vi "GetMainSequence.vi"(6 "Stepnum":i32, 8 "error in (no error)":errorcluster, 11 "Compiler Settings":T1={"Python Path"=path "", "Main File"="mainscript.py", "Meta File"="metascript.txt", "Aux File"="auxscript.py", "Pre File"="metascript.txt"}) -> (0 "error out":errorcluster, 3 "Main pulse":T2)   [LabVIEW 2019]
uses:
  PulseControl.ctl
  Compiler/Params.ctl
  PulseCompiler/CompilerSettings.ctl
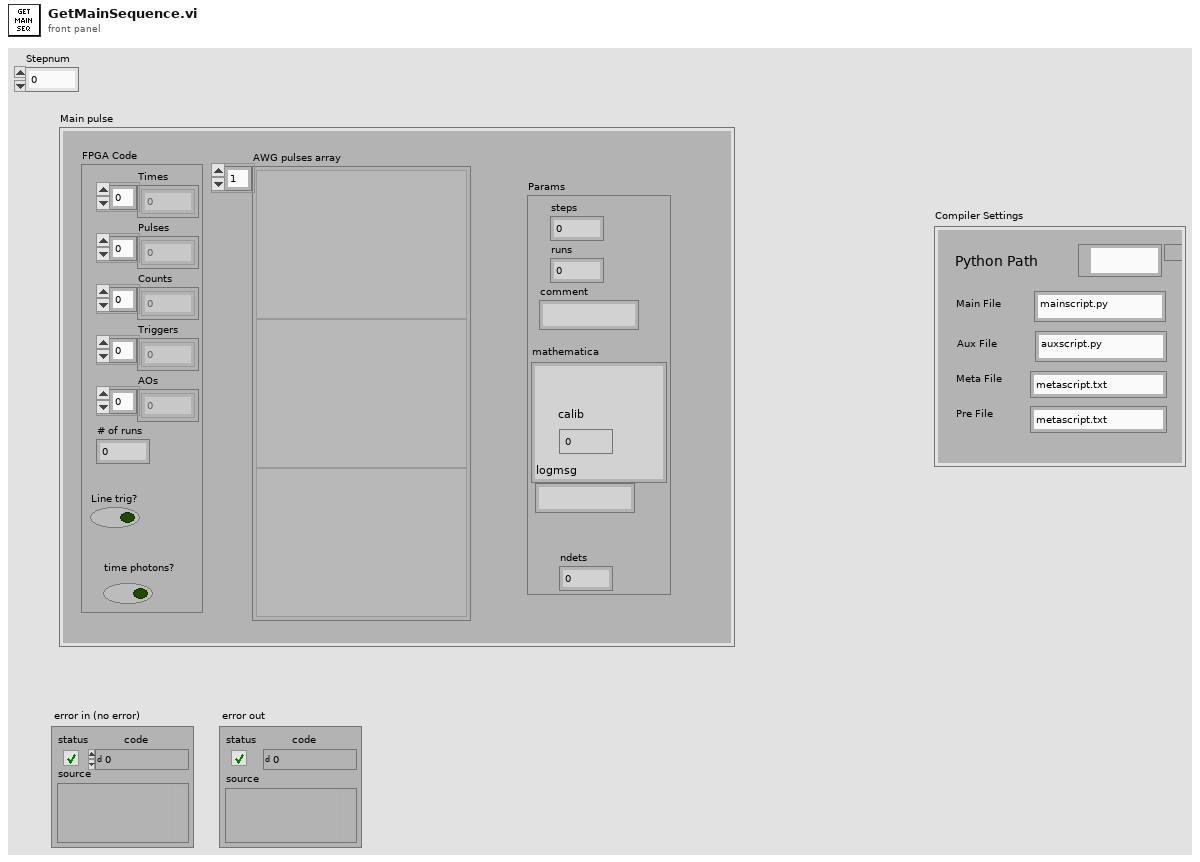
[diagram p1: front panel]
types:
  T1 = typedef "CompilerSettings.ctl" = cluster{"Python Path":path, "Main File":string, "Meta File":string, "Aux File":string, "Pre File":string}
  T2 = typedef "PulseControl.ctl" = cluster{"FPGA Code":cluster{"Times":u32[], "Pulses":u64[], "Counts":u8[], "Triggers":u8[], "AOs":u8[], "# of runs":i32, "Line trig?":bool, "time photons?":bool}, "AWG pulses array":variant[], "Params":T3}
  T3 = typedef "Params.ctl" = cluster{"steps":i16, "runs":i16, "comment":string, "mathematica":string, "calib":i8, "logmsg":string, "ndets":i16}
  T4 = typedef "SinglePulse.ctl" = cluster{"enabled":bool, "string":string, "time":dbl, "step":dbl, "dio":dbl, "count":dbl, "trigger":dbl, "AO":dbl}
  T5 = cluster{u32[], dbl[], "Count":dbl[], dbl[], dbl[], "# of runs":i32, "Line trig":bool, "save photon times":bool}
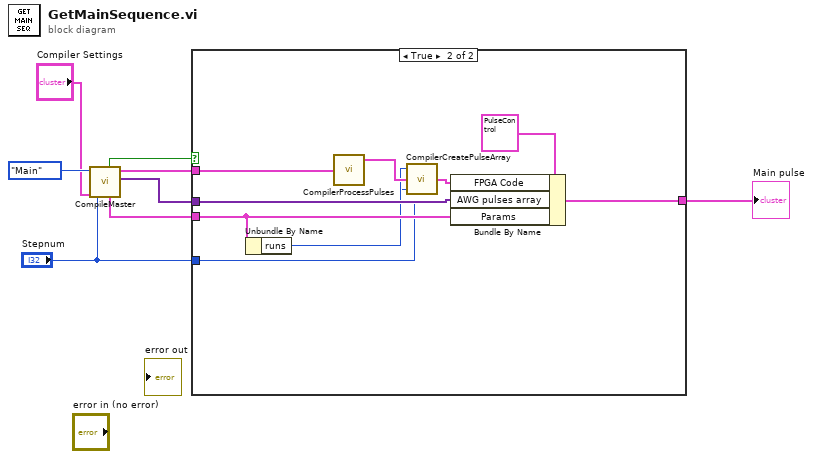
[diagram p0: block diagram]
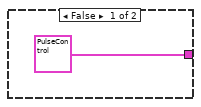
[diagram p2: hidden frame]
diagram:
  n1 = call "CompileMaster.vi"("Type"=enum16{"Meta", "Aux", "Main"}."Main" ("Enum"), "Stepnum"="Stepnum", "Compiler Settings"="Compiler Settings") -> ("CompileSuccess?"=w8:bool, "Params"=w7:T3, "PulseList"=w5:T4[], "RF Array"=w4:variant[])  [unwired: 1 in, 2 out]
  n2 = case shown="True" w8 {
    tunnel: [T2 {"FPGA Code"={"Times"=[], "Pulses"=[], "Counts"=[], "Triggers"=[], "AOs"=[], "# of runs"=0, "Line trig?"=FALSE, "time photons?"=FALSE}, "AWG pulses array"=[], "Params"={"steps"=0, "runs"=0, "comment"="", "mathematica"="", "calib"=0, "logmsg"="", "ndets"=0}} ("Pulse") w18] -> w3
    tunnel: w4 -> [_ w17]
    tunnel: w5 -> [_ w14]
    tunnel: w7 -> [_ w13]
    tunnel: "Stepnum" -> [_ w10]
    frame False {
    }
    frame True {
      n3 = Unbundle By Name(w13) -> ("runs"=w12:i16)
      n4 = call "CompilerProcessPulses.vi"("Pulse Seq In"=w14) -> ("Pulse Seq Out"=w16:T4[])  [unwired: 2 out]
      n5 = call "CompilerCreatePulseArray.vi"("step #"=w10, "Pulse Seq In"=w16, "runs"=w12) -> ("Pulse Seq Out"=w15:T5)
      n6 = Bundle By Name(cluster=T2 {"FPGA Code"={"Times"=[], "Pulses"=[], "Counts"=[], "Triggers"=[], "AOs"=[], "# of runs"=0, "Line trig?"=FALSE, "time photons?"=FALSE}, "AWG pulses array"=[], "Params"={"steps"=0, "runs"=0, "comment"="", "mathematica"="", "calib"=0, "logmsg"="", "ndets"=0}} ("Aux Pulse 2"), "FPGA Code"=w15, "AWG pulses array"=w17, "Params"=w13) -> (w18:T2)
    }
  }
  "Main pulse" <- w3
